vi "Configuracao.Variaveis.vi"() -> ()   [LabVIEW 2019]
panel:
  in  "PortaCOM":refnum<visa-resource-name>
  in  "EnderecoSerial":u8=1
  in  "TaxaComunicSerial":u32=9600
  in  "Paridade":u16(ring)=2 items=["None", "Ímpar", "Par", "Mark", "Space"]
  in  "TabelaPosicoesMemoria":string[][](array[string])
  in  "AceleracaoMaxInversor":dbl
  in  "ModeloInversor":string
  in  "AceleracaoMaxMotor":dbl
  in  "PotenciaMotor(W)":dbl
  in  "RotacaoMaxMotor(RPM)":dbl
  in  "ModeloMotor":string
  # "Inversor"
  # "Motor"
  # "Comunicacao"
  # "Endereço serial\nPorta COM \nTaxa de comunicação serial\nParidade\n     parity (even): paridade (par)\n     parity (odd): paridade (ímpar)"
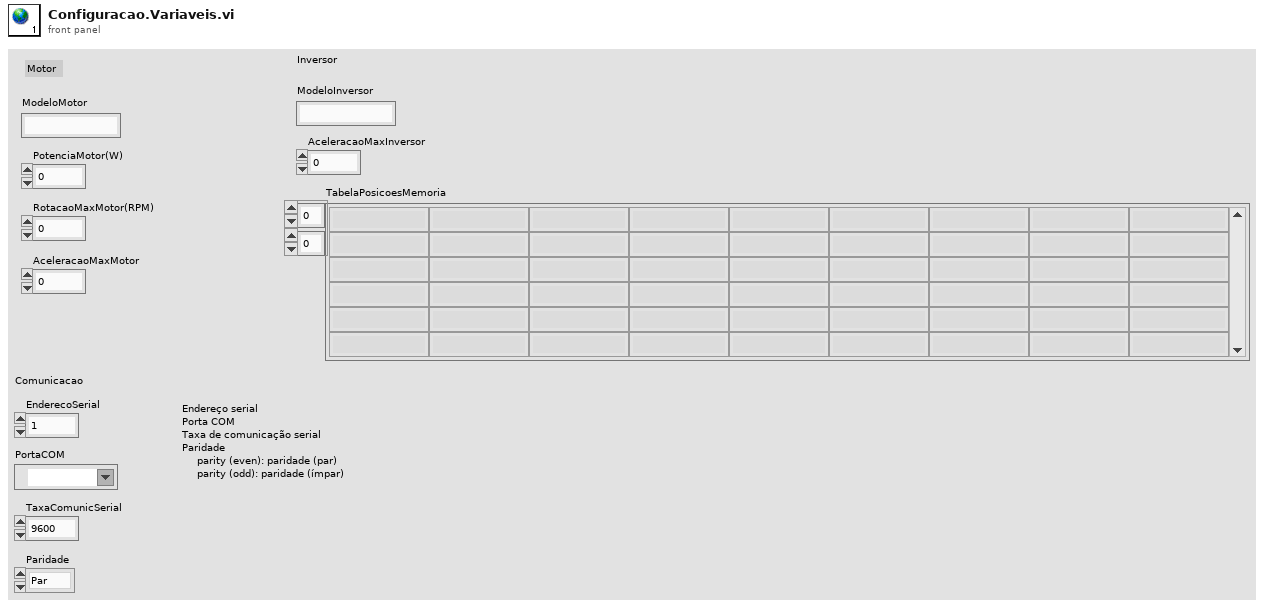
[diagram p1: front panel]
diagram:
